vi "Extract Error Codes From Files.vi"() -> ()   [LabVIEW 2009]
panel:
  out "Ring error":errorcluster
  in  "Ring":i32(ring)
  in  "Language":string="English"
  out "Files found/used":path[](array[path])
  out "Top path":path
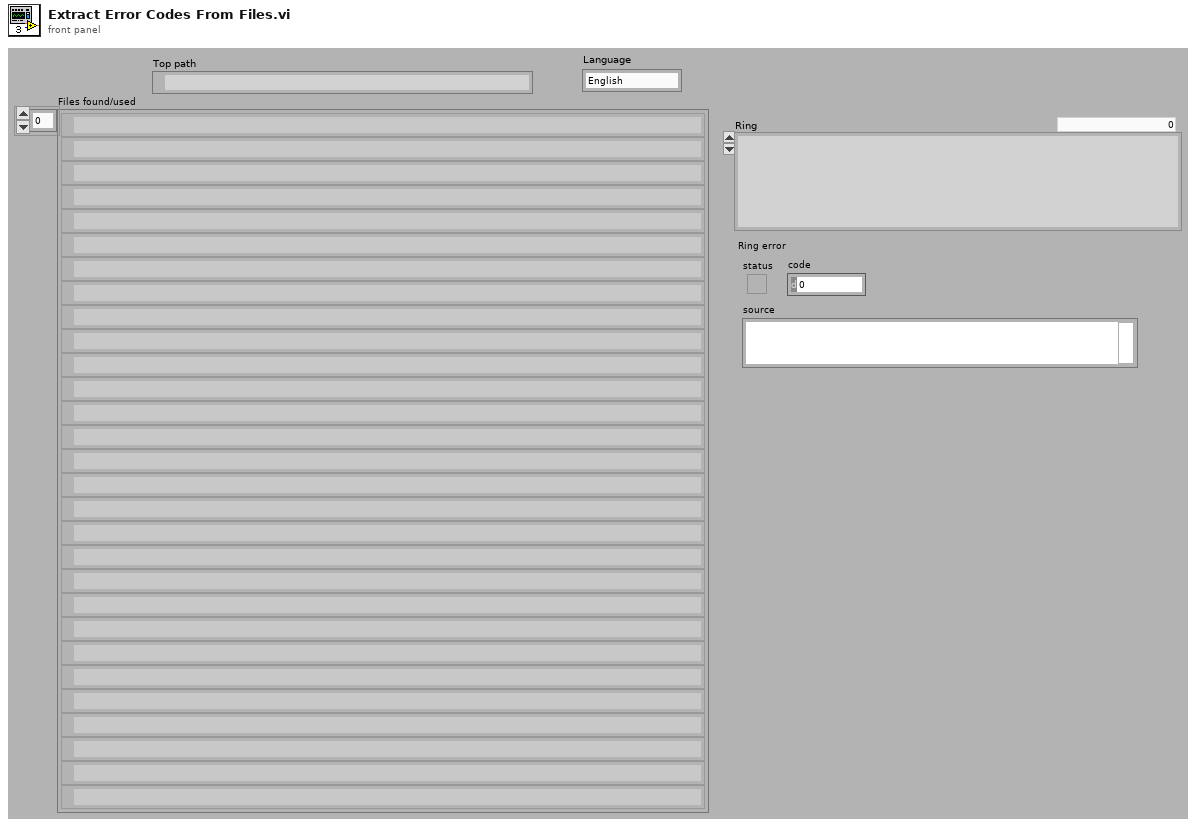
[diagram p1: front panel]
types:
  T1 = enum16{"open", "open or create", "create or replace", "create", "open (read only)"}
  T2 = typedef "LVStringsAndValuesArrayTypeDef.ctl" = cluster{"String":string, "Value":i32}[]
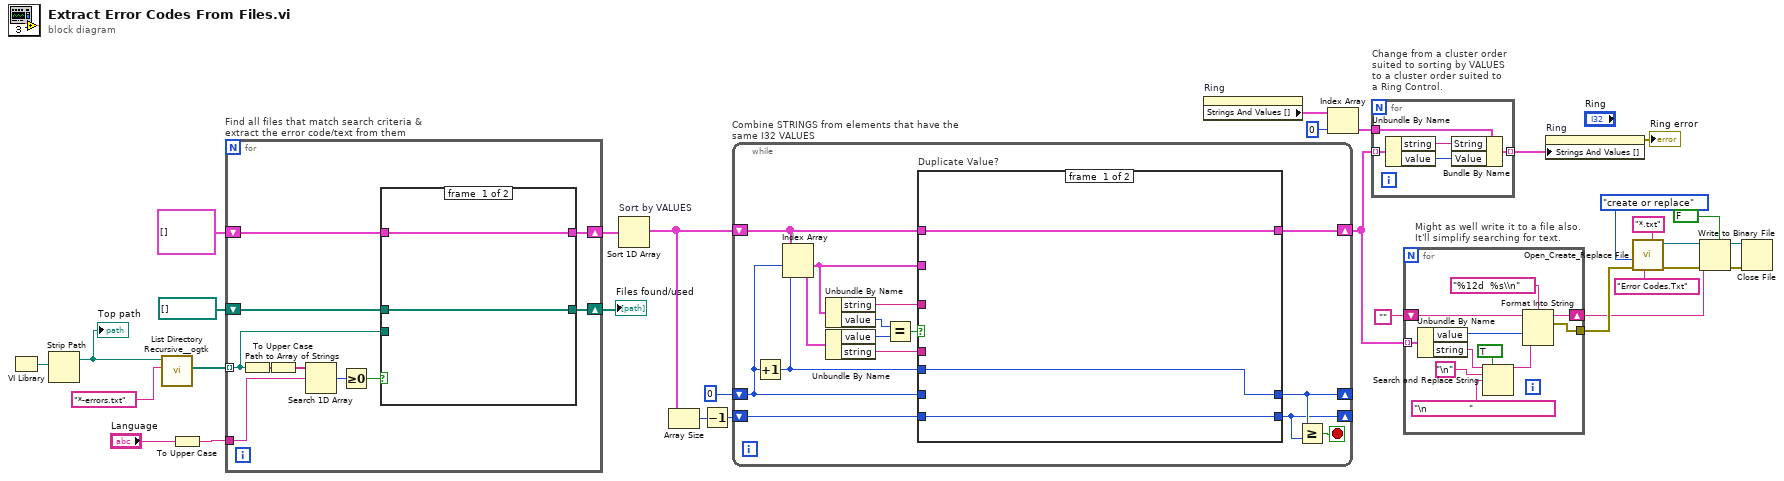
[diagram p0: block diagram]
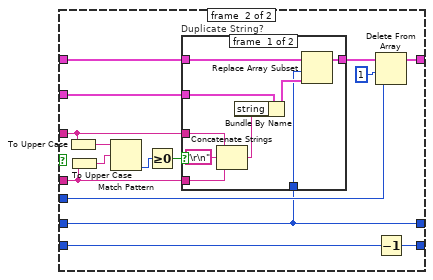
[diagram p2: hidden frame]
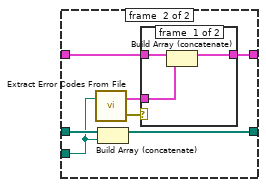
[diagram p4: hidden frame]
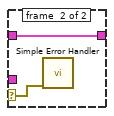
[diagram p5: hidden frame]
diagram:
  n1 = VI Library() -> (path=w31:path)
  n2 = Strip Path(path=w31) -> (stripped path=w29:path)  [unwired: 1 out]
  "Top path" <- w29
  n3 = call "List Directory Recursive__ogtk.vi"("pattern"="*-errors.txt", "Path"=w29) -> ("file paths"=w28:path[])  [unwired: 6 in, 3 out]
  n4 = To Upper Case(1:"Language") -> (0:w25:string)
  n5 = for "Find all files that match search criteria & extract the error code/text from them" {
    tunnel: w28 -> [w35] mode=indexing
    shift-right: [w34] -> w24
    shift-left: path[] [] ("file paths") -> [w36]
    tunnel: w25 -> [w39]
    shift-right: [w32] -> w22
    shift-left: cluster{"value":i32, "string":string}[] [] ("Array") -> [w33]
    n6 = Path to Array of Strings(0:w35) -> (2:w41:string[])  [unwired: 1 out]
    n7 = To Upper Case(1:w41) -> (0:w40:string[])
    n8 = Search 1D Array(1D array=w40, element=w39) -> (index of element=w38:i32)  [unwired: 1 in]
    n9 = Greater Or Equal To 0?(x=w38) -> (x >= 0?=w37:bool)
    n10 = case shown="True" w37 {
      tunnel: w36 -> [w43 w50]
      tunnel: w35 -> [_ w48]
      tunnel: [w43 w49] -> w34
      tunnel: w33 -> [w42 w47]
      tunnel: [w42 w45] -> w32
      frame #0 {
      }
      frame #1 {
        n11 = call "Extract Error Codes From File.vi"("XML File Path"=w48) -> ("error out"=w44:errorcluster, "Array"=w46:cluster{"value":i32, "string":string}[])  [unwired: 1 in]
        n12 = Build Array (concatenate)(w50, w48) -> (w49:path[])
        n13 = case shown="Error" w44 {
          selector: w44 -> [_ w54]
          tunnel: w47 -> [w53 w55]
          tunnel: w46 -> [w52 _]
          tunnel: [w51 w55] -> w45
          frame #0 {
            n14 = Build Array (concatenate)(w53, w52) -> (w51:cluster{"value":i32, "string":string}[])
          }
          frame #1 {
            n15 = call <vilib>:"Simple Error Handler.vi"("error in (no error)"=w54) -> ()  [unwired: 4 in, 5 out]
          }
        }
      }
    }
  }
  "Files found/used" <- w24
  n16 = Sort 1D Array "Sort by VALUES"(array=w22) -> (sorted array=w20:cluster{"value":i32, "string":string}[])
  n17 = Array Size(array=w20) -> (size(s)=w19:i32)
  n18 = Decrement(x=w19) -> (x-1=w17:i32)
  n19 = while "Combine STRINGS from elements that have the same I32 VALUES" {
    shift-right: [w64] -> w12
    shift-left: w20 -> [w66]
    shift-right: [w58] -> _
    shift-left: 0 -> [w63]
    shift-right: [w57] -> _
    shift-left: w17 -> [w65]
    stop <- w56 stop-if-true
    n20 = Increment(x=w63) -> (x+1=w62:i32)
    n21 = Index Array(array=w66, index #1=w63, index #2=w62) -> (element #1=w59:cluster{"value":i32, "string":string}, element #2=w70:cluster{"value":i32, "string":string})
    n22 = Unbundle By Name(w59) -> ("string"=w61:string, "value"=w69:i32)
    n23 = Unbundle By Name(w70) -> ("value"=w68:i32, "string"=w60:string)
    n24 = Equal?(x=w69, y=w68) -> (x = y?=w67:bool)
    n25 = case "Duplicate Value?" shown="True" w67 {
      tunnel: w66 -> [w73 w88]
      tunnel: w65 -> [w72 w87]
      tunnel: [w72 w86] -> w57
      tunnel: [w73 w85] -> w64
      tunnel: w63 -> [_ w80]
      tunnel: [w71 w80] -> w58
      tunnel: w62 -> [w71 w84]
      tunnel: w61 -> [_ w79]
      tunnel: w60 -> [_ w77]
      tunnel: w59 -> [_ w81]
      frame #0 {
      }
      frame #1 {
        n26 = To Upper Case(1:w79) -> (0:w78:string)
        n27 = To Upper Case(1:w77) -> (0:w76:string)
        n28 = Match Pattern(string=w78, regular expression=w76) -> (offset past match=w74:i32)  [unwired: 1 in, 3 out]
        n29 = Greater Or Equal To 0?(x=w74) -> (x >= 0?=w75:bool)
        n30 = case "Duplicate String?" shown="False" w75 {
          tunnel: w88 -> [w97 w98]
          tunnel: [w96 w98] -> w82
          tunnel: w81 -> [w93 _]
          tunnel: w80 -> [w91 _]
          tunnel: w79 -> [w90 _]
          tunnel: w77 -> [w89 _]
          frame #0 {
            n31 = Concatenate Strings(w90, "\r\n", w89) -> (w94:string)
            n32 = Bundle By Name(cluster=w93, "string"=w94) -> (w92:cluster{"value":i32, "string":string})
            n33 = Replace Array Subset(array=w97, new element=w92, index=w91) -> (w96:cluster{"value":i32, "string":string}[])
          }
          frame #1 {
          }
        }
        n34 = Delete From Array(array=w82, length=1, index=w84) -> (array with subset deleted=w85:cluster{"value":i32, "string":string}[])  [unwired: 1 out]
        n35 = Decrement(x=w87) -> (x-1=w86:i32)
      }
    }
    n36 = Greater Or Equal?(x=w58, y=w57) -> (x >= y?=w56:bool)
  }
  n37 = property on="Ring" class="Ring (strict)"() -> ("Strings And Values []"=w16:T2)  [unwired: 2 in, 2 out]
  n38 = Index Array(array=w16, index=0) -> (element=w14:cluster{"String":string, "Value":i32})
  n39 = for "Change from a cluster order\nsuited to sorting by VALUES \nto a cluster order suited to\na Ring Control." {
    tunnel: w12 -> [w103] mode=indexing
    tunnel: w14 -> [w102]
    tunnel: [w99] -> w13 mode=indexing
    n40 = Unbundle By Name(w103) -> ("string"=w101:string, "value"=w100:i32)
    n41 = Bundle By Name(cluster=w102, "String"=w101, "Value"=w100) -> (w99:cluster{"String":string, "Value":i32})
  }
  n42 = for "Might as well write it to a file also.\nIt'll simplify searching for text." {
    tunnel: w12 -> [w114] mode=indexing
    shift-right: [w113] -> w4
    shift-left: "" -> [w112]
    tunnel: [w104] -> w5
    n43 = Unbundle By Name(w114) -> ("value"=w110:i32, "string"=w109:string)
    n44 = Search and Replace String(replace all?=TRUE ("replace all? (F)"), input string=w109, search string="\n", replace string="\n              " ("search string")) -> (result string=w108:string)  [unwired: 4 in, 3 out]
    n45 = Format Into String(format string="%12d  %s\\n", initial string=w112, w110, w108) -> (resulting string=w113:string, error out=w104:errorcluster)  [unwired: 1 in]
  }
  n46 = property on="Ring" class="Ring (strict)"("Strings And Values []"=w13) -> (error out=→"Ring error":errorcluster)  [unwired: 2 in, 1 out]
  n47 = call <vilib>:"Open_Create_Replace File.vi"("pattern"="*.txt", "default name"="Error Codes.Txt", "error in (no error)"=w5, "function (open:0)"=T1."create or replace") -> ("error out"=w9:errorcluster, "refnum"=w10:refnum<file>)  [unwired: 4 in, 2 out]
  n48 = Write to Binary File(file (use dialog)=w10, data=w4, error in=w9, 5:FALSE ("prepend array or string size? (T)")) -> (refnum out=w2:refnum<file>, error out=w3:errorcluster)  [unwired: 2 in, 1 out]
  n49 = Close File(refnum=w2, error in=w3) -> ()  [unwired: 2 out]
